vi "Form Clumps.vi"(8 "error in (no error)":errorcluster, 11 "Clump Precursors":T1[](array[typedef]) {"Channels"."Mapping"."VS Reference" format="%.0x"}) -> (0 "error out":errorcluster, 3 "Clumps":T8[](array[typedef]))   [LabVIEW 2021]
uses:
  <vilib>/NI VeriStand/Custom Device API/Custom Device Channel Type.ctl
  <vilib>/NI VeriStand/Custom Device API/Custom Device API.lvlib
  System Explorer/SubVIs/Modbus Type.ctl
  Shared/Modbus Master Shared.lvlib
  clump.ctl
  Clump Precursor.ctl
  Shared/Controls/Data Model/DataType.ctl
  <vilib>/NI VeriStand/Custom Device API/Custom Device Item Ref.ctl
  Shared/Controls/Data Model/Mapping.ctl
  Shared/Controls/Data Model/Channel.ctl
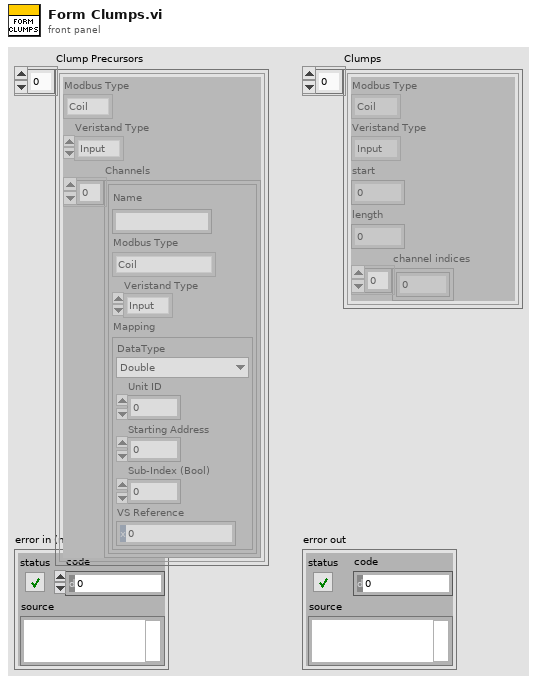
[diagram p1: front panel]
types:
  T1 = typedef "Modbus Master Shared.lvlib/Clump Precursor.ctl" = cluster{"Modbus Type":T2, "Veristand Type":T3, "Channels":T4[]}
  T2 = typedef "Modbus Master Shared.lvlib/Modbus Type.ctl" = enum16{"Coil", "Discrete Input", "Holding Register", "Input Register"}
  T3 = typedef "Custom Device API.lvlib/Custom Device Channel Type.ctl" = enum16{"Input", "Output"}
  T4 = typedef "Modbus Master Shared.lvlib/Channel.ctl" = cluster{"Name":string, "Modbus Type":T2, "Veristand Type":T3, "Mapping":T5}
  T5 = typedef "Modbus Master Shared.lvlib/Mapping.ctl" = cluster{"DataType":T6, "Unit ID":u8, "Starting Address":u16, "Sub-Index (Bool)":u16, "VS Reference":T7}
  T6 = typedef "Modbus Master Shared.lvlib/DataType.ctl" = enum16{"Double", "Single", "I64", "I32", "I16", "I8", "U64", "U32", "U16", "U8", "Boolean"}
  T7 = typedef "Custom Device API.lvlib/Custom Device Item Ref.ctl" = u64
  T8 = typedef "Modbus Master Shared.lvlib/clump.ctl" = cluster{"Modbus Type":T2, "Veristand Type":T3, "start":i32, "length":i32, "channel indices":i32[]}
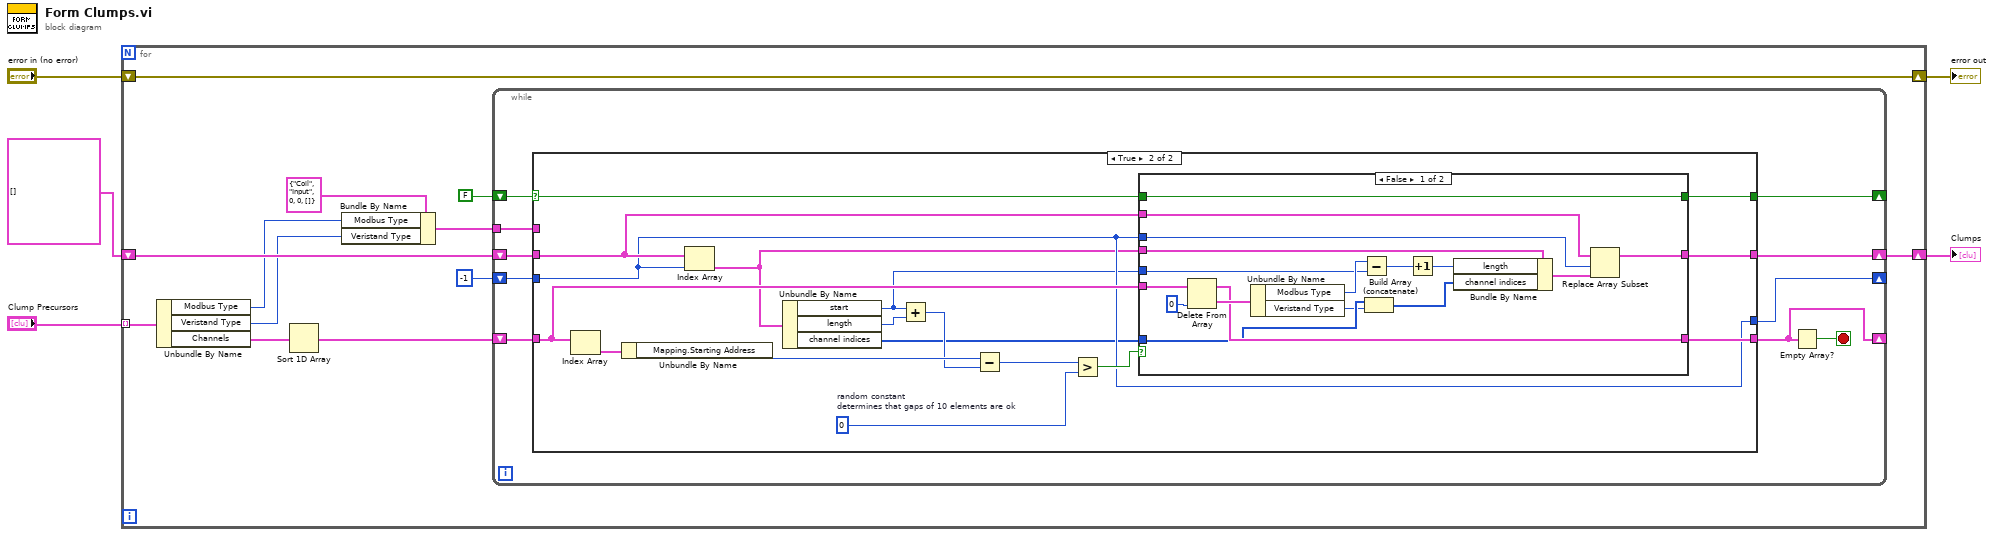
[diagram p0: block diagram]
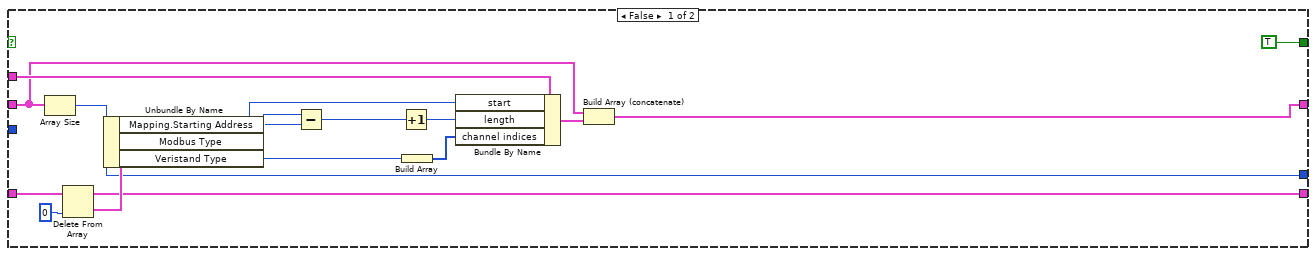
[diagram p2: hidden frame]
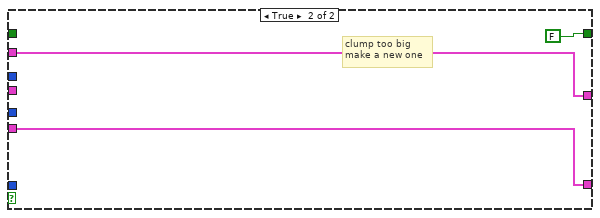
[diagram p3: hidden frame]
diagram:
  n1 = for {
    tunnel: "Clump Precursors" -> [w17] mode=indexing
    shift-right: [w6] -> w2
    shift-left: "error in (no error)" -> [w6]
    shift-right: [w14] -> w5
    shift-left: T8[] [] -> [w15]
    n2 = Unbundle By Name(w17) -> ("Modbus Type"=w11:T2, "Veristand Type"=w12:T3, "Channels"=w16:T4[])
    n3 = Sort 1D Array(array=w16) -> (sorted array=w10:T4[])
    n4 = Bundle By Name(cluster=T8 {"Modbus Type"=enum."Coil", "Veristand Type"=enum."Input", "start"=0, "length"=0, "channel indices"=[]} ("output cluster"), "Modbus Type"=w11, "Veristand Type"=w12) -> (w9:T8)
    n5 = while {
      shift-right: [w22] -> _
      shift-left: w10 -> [w23]
      shift-right: [w24] -> w14
      shift-left: w15 -> [w25]
      shift-right: [w26] -> _
      shift-left: FALSE -> [w27]
      tunnel: w9 -> [w20]
      shift-right: [w18] -> _
      shift-left: -1 -> [w19]
      stop <- w21 stop-if-true
      n6 = case shown="True" w27 {
        selector: w27 -> [_ w53]
        tunnel: [TRUE w52] -> w26
        tunnel: w25 -> [w33 w49]
        tunnel: [w35 w48] -> w24
        tunnel: [w37 w51] -> w22
        tunnel: w23 -> [w43 w50]
        tunnel: w20 -> [w36 _]
        tunnel: w19 -> [_ w47]
        tunnel: [w32 w47] -> w18
        frame False {
          n7 = Array Size(array=w33) -> (size(s)=w32:i32)
          n8 = Delete From Array(array=w43, index=0) -> (deleted portion=w42:T4, array with subset deleted=w37:T4[])  [unwired: 1 in]
          n9 = Unbundle By Name(w42) -> ("Mapping.Starting Address"=w40:u16, "Modbus Type"=w41:T2, "Veristand Type"=w29:T3)
          n10 = Subtract(x=w41, y=w40) -> (x-y=w39:u16)
          n11 = Increment(x=w39) -> (x+1=w38:u16)
          n12 = Build Array(w29) -> (w28:T3[])
          n13 = Bundle By Name(cluster=w36, "start"=w40, "length"=w38, "channel indices"=w28) -> (w34:T8)
          n14 = Build Array (concatenate)(w33, w34) -> (w35:T8[])
        }
        frame True {
          w55 = 0  # random constant determines that gaps of 10 elements are ok
          n15 = Index Array(array=w50) -> (element=w59:T4)  [unwired: 1 in]
          n16 = Unbundle By Name(w59) -> ("Mapping.Starting Address"=w58:u16)
          n17 = Index Array(array=w49, index=w47) -> (element=w46:T8)
          n18 = Unbundle By Name(w46) -> ("start"=w45:i32, "length"=w60:i32, "channel indices"=w44:i32[])
          n19 = Add(x=w45, y=w60) -> (x+y=w57:i32)
          n20 = Subtract(x=w58, y=w57) -> (x-y=w56:i32)
          n21 = Greater?(x=w56, y=w55) -> (0:w54:bool)
          n22 = case shown="False" w54 {
            tunnel: w53 -> [w66 _]
            tunnel: [w66 FALSE] -> w52
            tunnel: [w69 w80] -> w51
            tunnel: w50 -> [w70 w80]
            tunnel: w49 -> [w77 w79]
            tunnel: [w76 w79] -> w48
            tunnel: w47 -> [w75 _]
            tunnel: w46 -> [w67 _]
            tunnel: w45 -> [w65 _]
            tunnel: w44 -> [w63 _]
            frame False {
              n23 = Delete From Array(array=w70, index=0) -> (deleted portion=w74:T4, array with subset deleted=w69:T4[])  [unwired: 1 in]
              n24 = Unbundle By Name(w74) -> ("Modbus Type"=w73:T2, "Veristand Type"=w62:T3)
              n25 = Subtract(x=w73, y=w65) -> (x-y=w72:i32)
              n26 = Build Array (concatenate)(w63, w62) -> (w61:i32[])
              n27 = Increment(x=w72) -> (x+1=w71:i32)
              n28 = Bundle By Name(cluster=w67, "length"=w71, "channel indices"=w61) -> (w68:T8)
              n29 = Replace Array Subset(array=w77, new element=w68, index=w75) -> (w76:T8[])
            }
            frame True {
              # "clump too big\nmake a new one"
            }
          }
        }
      }
      n30 = Empty Array?(array=w22) -> (empty?=w21:bool)
    }
  }
  "Clumps" <- w5
  "error out" <- w2
